vi "4 probe data v1.3.vi"() -> ()   [LabVIEW 2014]
uses:
  <vilib>/Analysis/baseanly.llb/Mean (DBL).vi
  <instrlib>/Keithley 24XX/Public/Data/Read (Single Point).vi
  <vilib>/MakerHub/LINX/Public/Peripherals/Analog/Analog Read 1 Chan.vi
  <instrlib>/Tektronix TDS 200 1000 2000 Series/Tektronix TDS 200 1000 2000 Series.lvlib
  <vilib>/MakerHub/LINX/LMH-LINX.lvlib
  <vilib>/Analysis/NI_AALBase.lvlib
  <instrlib>/Keithley 24XX/Keithley 24XX.lvlib
panel:
  out "Resistance-Time":sgl[](graph)
  out "Data IV Keithley":string
  in  "Data IV Keithley 2":path=path "c:/myfile.txt"
  out "IV Curve":cluster{sgl[], dbl[]}(graph)
  in  "Stop Voltage/Current":dbl=2.0
  in  "VISA resource name 2":refnum<visa-resource-name>="GPIB9::24::INSTR"
  in  "Serial Configuration 2":T1={"Baud Rate"=9600, "Parity"=0, "Data Bits"=8, "Stop Bits"=10, "Flow Control"=0} {"Flow Control" items=["None", "XON/XOFF", "RTS/CTS", "XON/XOFF & RTS/CTS", "DTR/DSR", "XON/XOFF & DTR/DSR"]; "Stop Bits" items=["1.0"=10, "1.5"=15, "2.0"=20]; "Data Bits" items=["7"=7, "8"=8]; "Parity" items=["None", "Odd", "Even", "Mark", "Space"]; "Baud Rate" items=["300"=300, "600"=600, "1200"=1200, "2400"=2400, "4800"=4800, "9600"=9600, "19200"=19200]}
  out "Voltage":sgl
  out "Current":sgl
  out "Resistance":sgl
  in  "Voltage Manual Range (1.0)":dbl=1.0
  in  "Current Manual Range (1.0)":dbl=1.0
  in  "Resistance Manual Range (1.0)":dbl=1.0
  in  "Enable Voltage Auto Range (T:Enable)":bool
  in  "Enable Current Auto Range (T:Enable)":bool=TRUE
  in  "Enable Resistance Auto Range (T:Enable)":bool
  in  "Compliance  Level (0.1)":dbl=1.0
  in  "Source Mode  (0: Voltage)":u16(ring) items=["Voltage", "Current"]
  in  "Step":dbl=1.0
  in  "current multiplier":dbl=1.0
  in  "Start Voltage/Current":dbl
  in  "Stop Button":bool
  out "Ard 4":dbl
  out "Ard 3":dbl
  out "Ard 2":dbl
  out "Ard 1":dbl
  out "Ard 0":dbl
  out "Data Ch4":string
  in  "Data Ch4":path=path "c:/myfile4.txt"
  out "Ard3-Osc4":cluster{"Y":dbl[], "Y":dbl[]}[](graph)
  out "Data Ch3":string
  in  "Data Ch3":path=path "c:/myfile3.txt"
  out "Ard2-Osc 3":cluster{"Y":dbl[], "Y":dbl[]}[](graph)
  out "Data Ch2":string
  in  "Data Ch2":path=path "c:/myfile2.txt"
  out "Ard1-Osc 2":cluster{"Y":dbl[], "Y":dbl[]}[](graph)
  out "Data Ch1":string
  in  "Data Ch1":path=path "c:/myfile1.txt"
  out "Ard0-Osc 1":cluster{"Y":dbl[], "Y":dbl[]}[](graph)
  out "Ch1":dbl
  out "Ch2":dbl
  out "Ch3":dbl
  out "Ch4":dbl
  out "Loop Rate (Hz)":u32
  out "Analog Data 4":dbl(graph)
  in  "AI Channel 4":u8=4
  in  "AI Channel 3":u8=3
  in  "AI Channel 2":u8=2
  in  "AI Channel 1":u8=1
  in  "AI Channel 0":u8
  in  "Serial Port":refnum<visa-resource-name>="COM6"
  in  "Channel 4 (3: Channel 4)":u16(ring)=3 items=["Channel 1", "Channel 2", "Channel 3", "Channel 4", "Math", "Reference A", "Reference B", "Reference C", "Reference D"]
  in  "Probe Attenuation 4 (0.1)":dbl=0.1
  in  "Vertical Coupling 4 (1: DC)":u16(ring)=1 items=["AC", "DC", "Ground"]
  in  "Channel 3 (2: Channel 3)":u16(ring)=2 items=["Channel 1", "Channel 2", "Channel 3", "Channel 4", "Math", "Reference A", "Reference B", "Reference C", "Reference D"]
  in  "Probe Attenuation 3 (0.1)":dbl=0.1
  in  "Vertical Coupling 3 (1: DC)":u16(ring)=1 items=["AC", "DC", "Ground"]
  in  "Channel 2 (1: Channel 2)":u16(ring)=1 items=["Channel 1", "Channel 2", "Channel 3", "Channel 4", "Math", "Reference A", "Reference B", "Reference C", "Reference D"]
  in  "Channel 1 (0: Channel 1)":u16(ring) items=["Channel 1", "Channel 2", "Channel 3", "Channel 4", "Math", "Reference A", "Reference B", "Reference C", "Reference D"]
  in  "Serial Configuration":T2={"Baud Rate"=9600, "Parity"=0, "Stop Bits"=10, "Flow Control"=2} {"Flow Control" items=["None", "XON/XOFF", "RTS/CTS", "XON/XOFF & RTS/CTS", "DTR/DSR", "XON/XOFF & DTR/DSR"]; "Stop Bits" items=["1.0"=10, "1.5"=15, "2.0"=20]; "Parity" items=["None", "Odd", "Even", "Mark", "Space"]; "Baud Rate" items=["300"=300, "600"=600, "1200"=1200, "2400"=2400, "4800"=4800, "9600"=9600, "19200"=19200]}
  in  "Probe Attenuation 2 (0.1)":dbl=0.1
  in  "Vertical Coupling 2 (1: DC)":u16(ring)=1 items=["AC", "DC", "Ground"]
  in  "Probe Attenuation 1 (0.1)":dbl=0.1
  in  "Vertical Coupling 1 (1: DC)":u16(ring)=1 items=["AC", "DC", "Ground"]
  in  "Timeout (10000 ms)":u32=500
  in  "VISA resource name":refnum<visa-resource-name>="USB0::0x0699::0x03A6::C044157::INSTR"
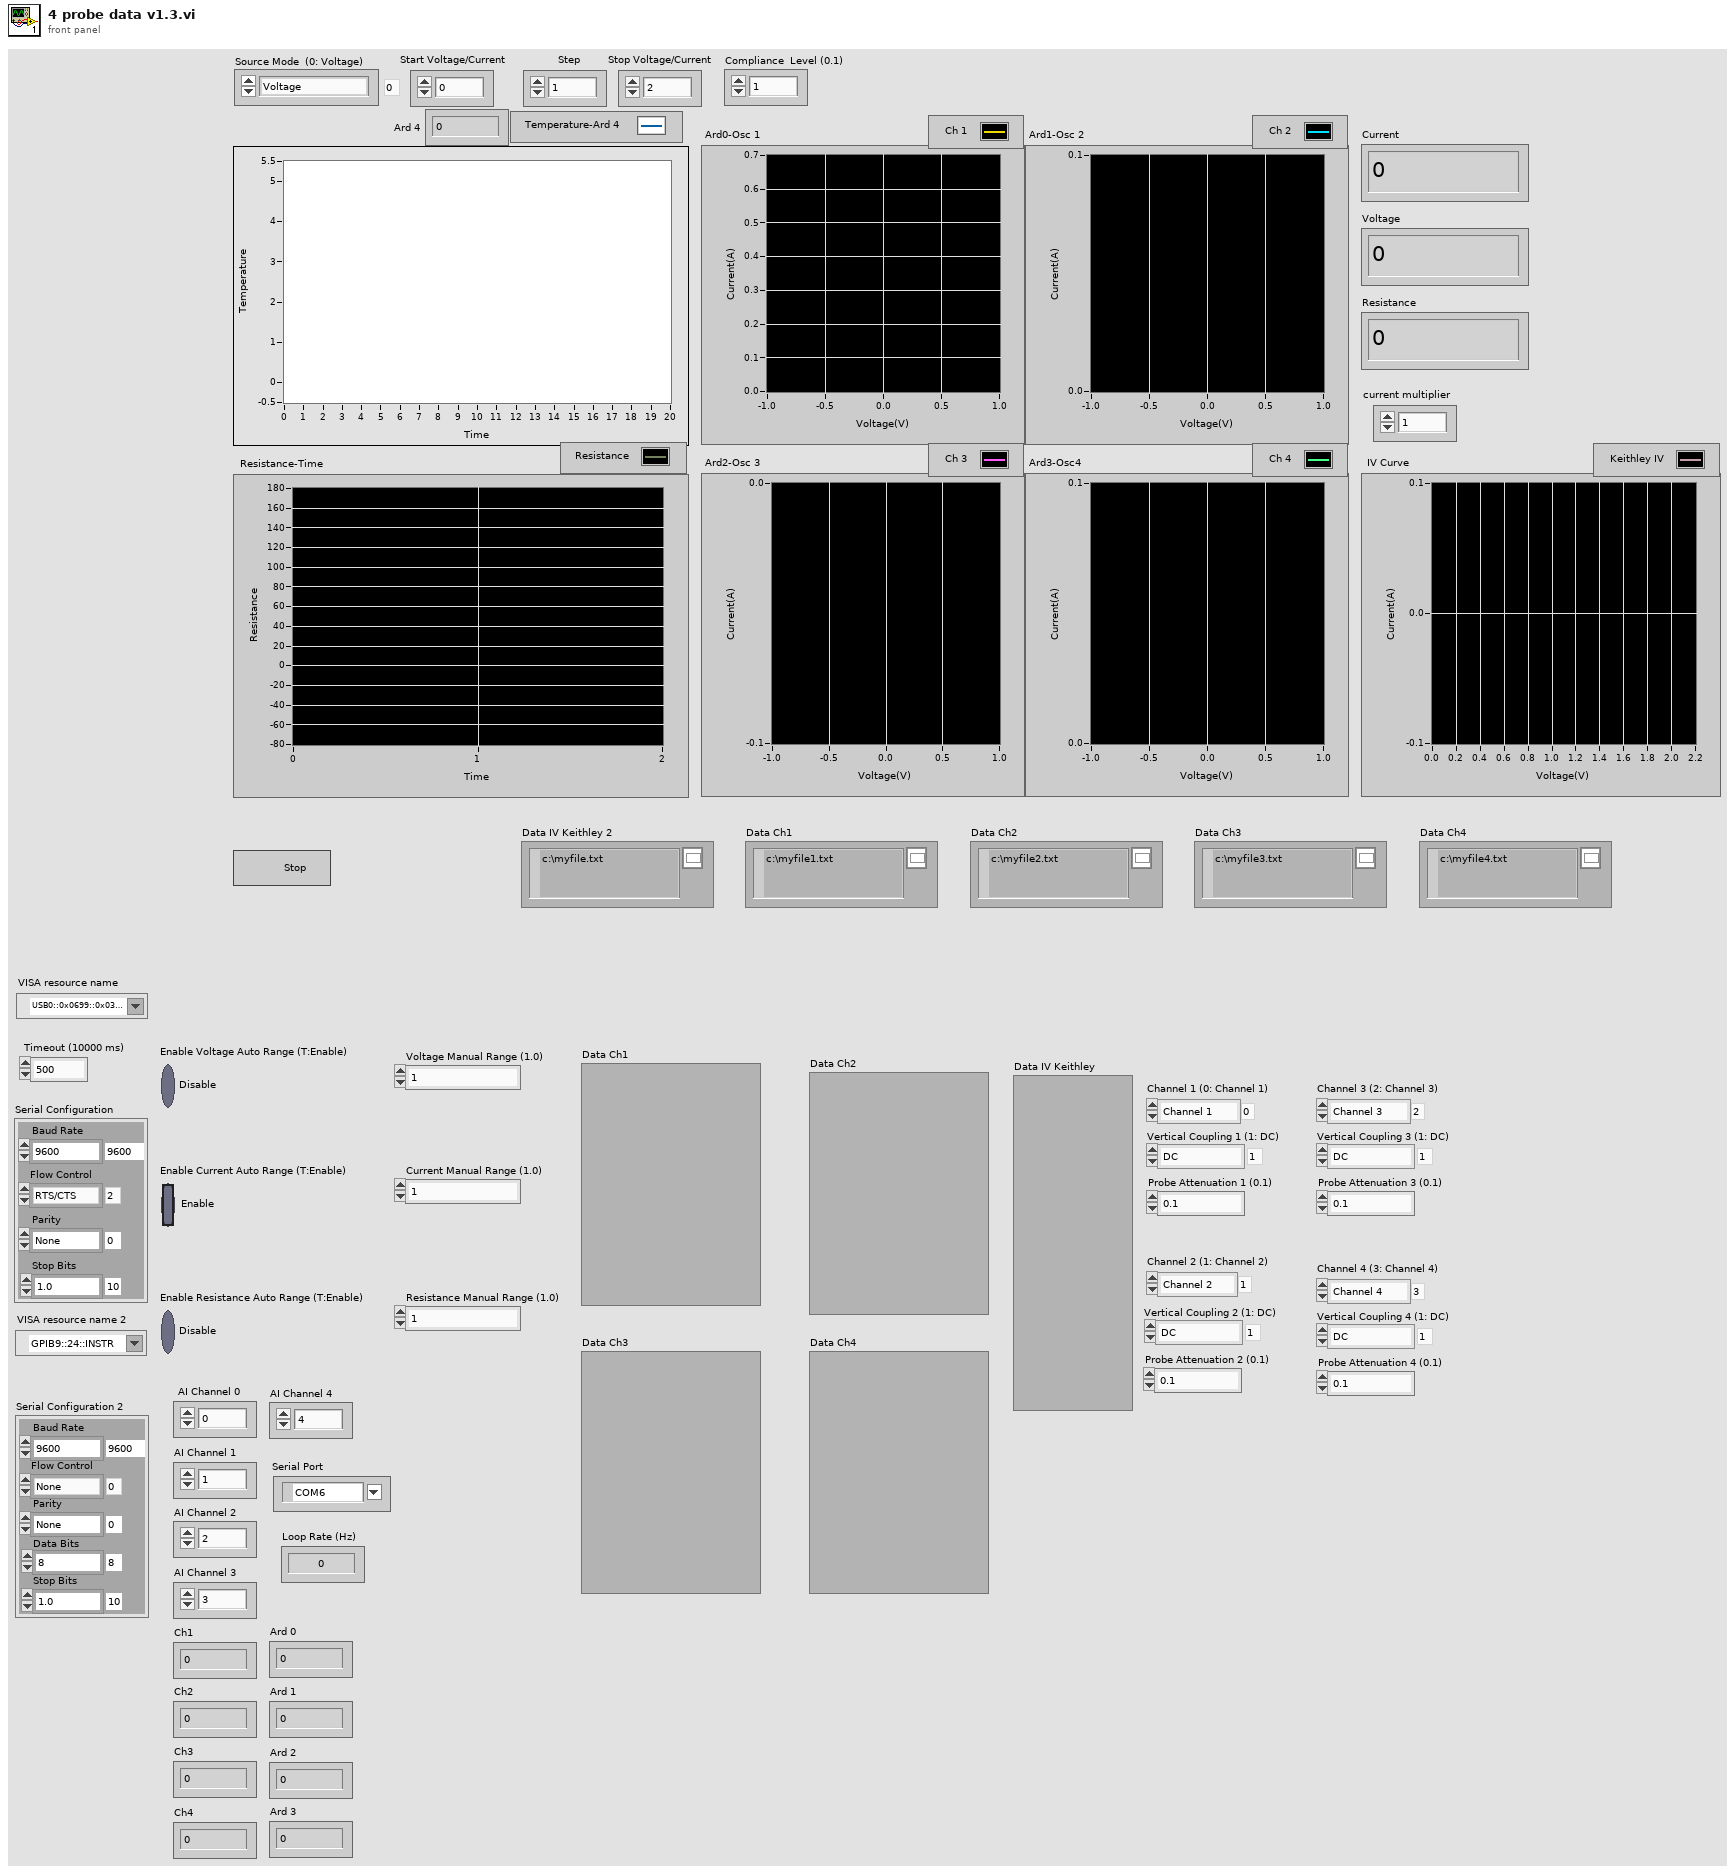
[diagram p1: front panel]
types:
  T1 = cluster{"Baud Rate":u32, "Parity":u16, "Data Bits":u16, "Stop Bits":u16, "Flow Control":u16}
  T2 = cluster{"Baud Rate":u32, "Parity":u16, "Stop Bits":u16, "Flow Control":u16}
  T3 = enum16{"open", "replace", "create", "open or create", "replace or create", "replace or create with confirmation"}
  T4 = typedef "LMH-LINX.lvlib/LINX Ref.ctl" = cluster{"Platform":T5, "Interface":T6, "LINX Device Config":T7}
  T5 = typedef "LMH-LINX.lvlib/Platform.ctl" = enum16{"LINX", "myRIO"}
  T6 = typedef "LMH-LINX.lvlib/Interface.ctl" = enum16{"Serial", "TCP"}
  T7 = typedef "LMH-LINX.lvlib/Device.lvlib/LINX Device Config.ctl" = cluster{"Interface":T6, "COM Port":refnum<visa-resource-name>, "TCP Configuration":T8, "Device Family":u8, "Device ID":u8, "Device Name":string, "TCP Ref":refnum<k5>, "Channels":T9}
  T8 = typedef "LMH-LINX.lvlib/Device.lvlib/TCP Config.ctl" = cluster{"IP Address":string, "Port":u16}
  T9 = typedef "LMH-LINX.lvlib/Channels.ctl" = cluster{"DI":u8[], "DO":u8[], "AI":u8[], "AO":u8[], "PWM":u8[], "QE":u8[], "UART":u8[], "I2C 2":u8[], "SPI":u8[], "CAN":u8[], "Servo":u8[], "AI Ref (V)":dbl, "AO Ref (V)":dbl, "AO Resolution (Bits)":u8}
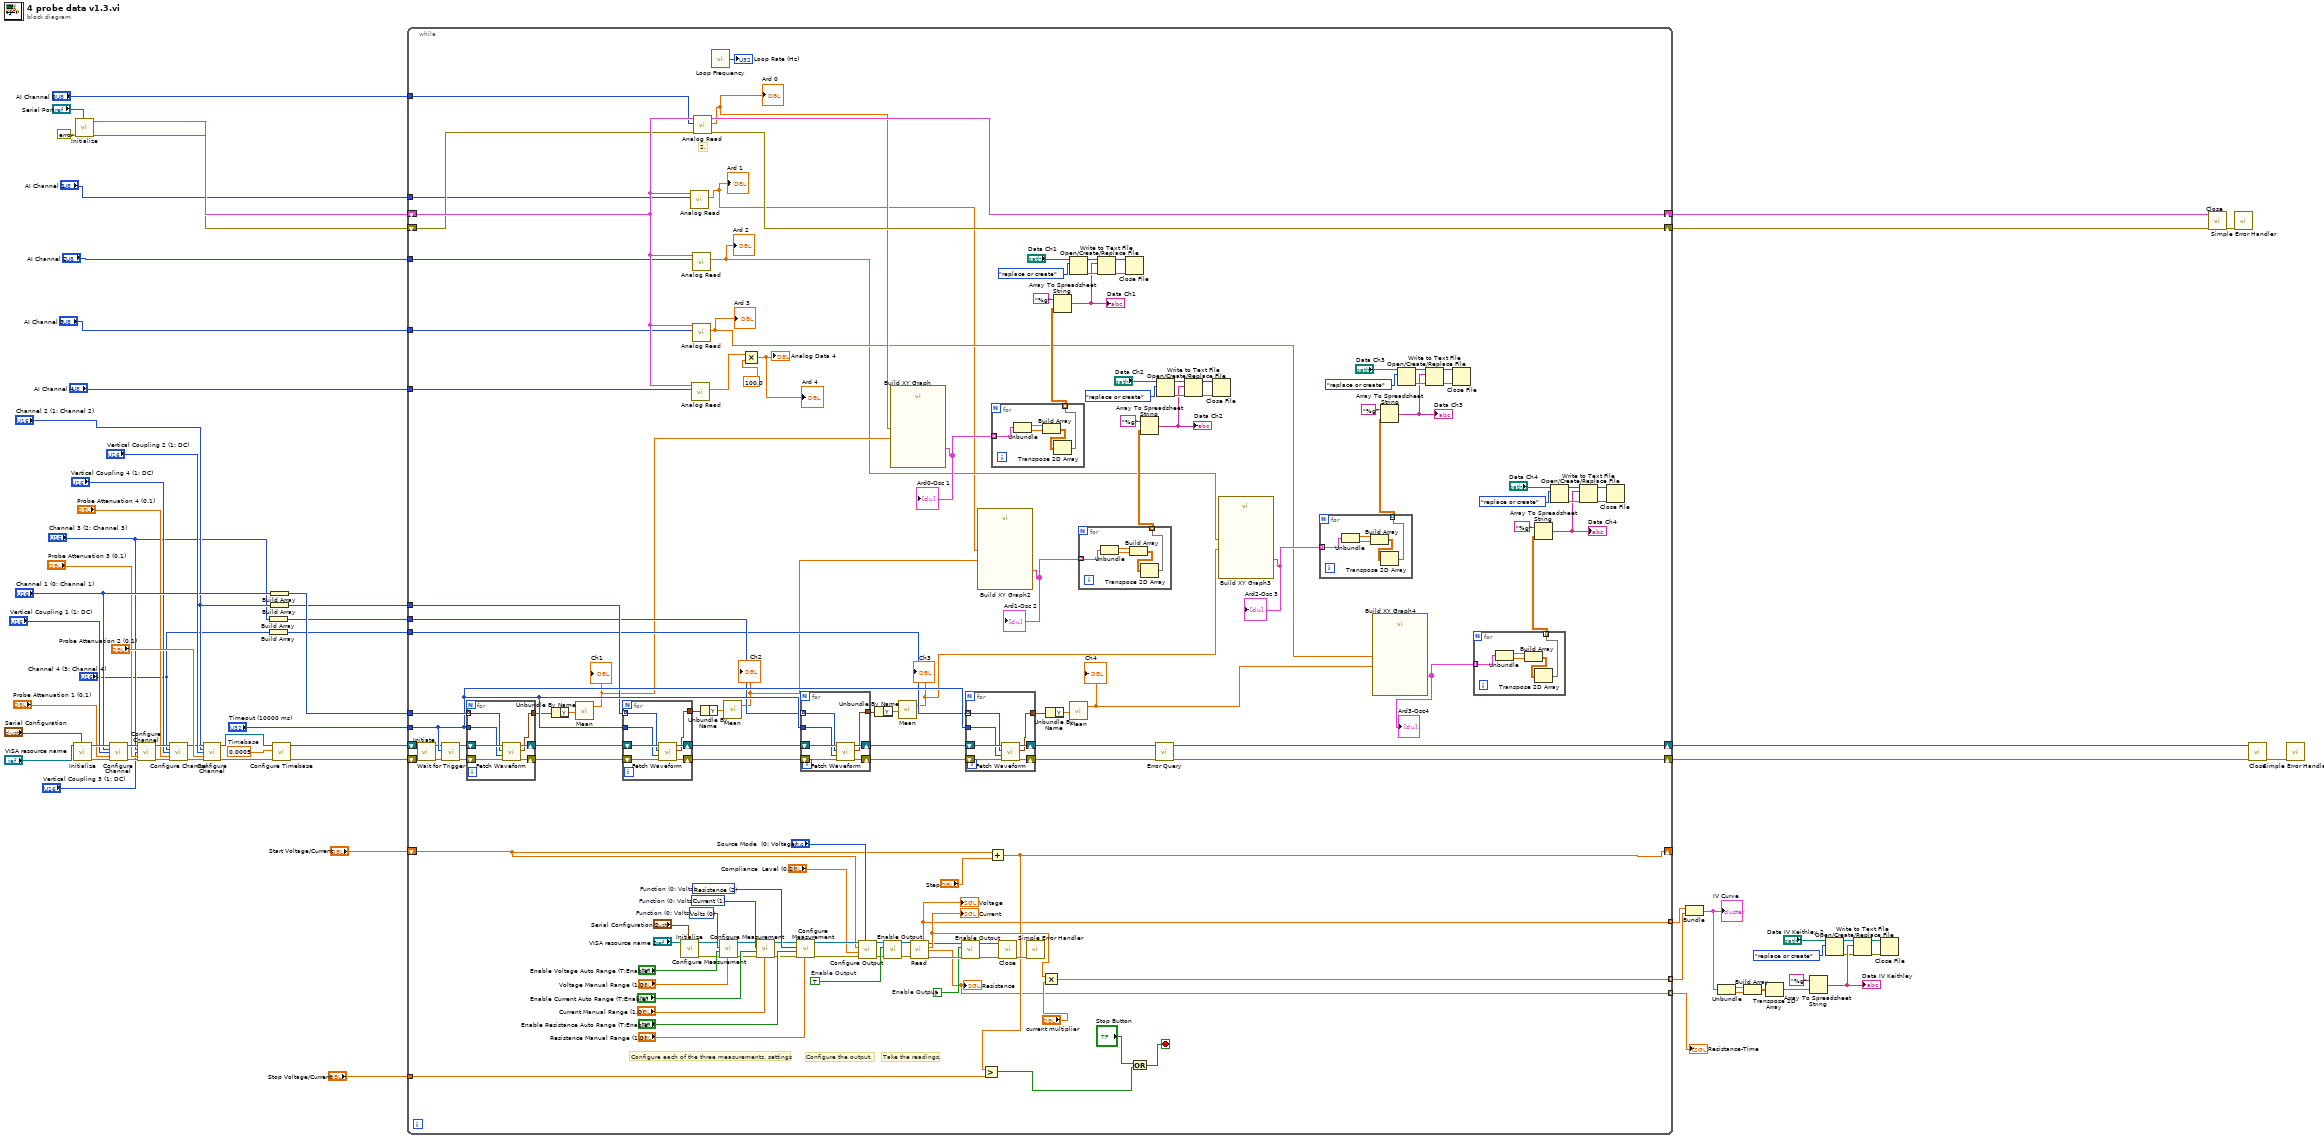
[diagram p0: block diagram]
diagram:
  w51 = 0.0005  # Timebase
  n1 = call <instrlib>:"Initialize.vi"("Serial Configuration"="Serial Configuration", "VISA resource name"="VISA resource name") -> ("error out"=w60:errorcluster, "VISA resource name out"=w61:refnum<visa-resource-name>)  [unwired: 3 in, 5 out]
  n2 = call <instrlib>:"Initialize.vi"("Serial Port"="Serial Port", "Error In"=errorcluster {"status"=FALSE, "code"=0, "source"=""}) -> ("Error Out"=w29:errorcluster, "LINX Ref"=w30:T4)  [unwired: 7 in, 1 out]
  n3 = call <instrlib>:"Configure Channel.vi"("VISA resource name"=w61, "Channel (0: Channel 1)"="Channel 1 (0: Channel 1)", "Vertical Coupling (1: DC)"="Vertical Coupling 1 (1: DC)", "Probe Attenuation (10: 10X)"="Probe Attenuation 1 (0.1)", "error in (no error)"=w60) -> ("VISA resource name out"=w46:refnum<visa-resource-name>, "error out"=w43:errorcluster)  [unwired: 4 in, 5 out]
  n4 = call <instrlib>:"Configure Channel.vi"("VISA resource name"=w46, "Channel (0: Channel 1)"="Channel 3 (2: Channel 3)", "Vertical Coupling (1: DC)"="Vertical Coupling 3 (1: DC)", "Probe Attenuation (10: 10X)"="Probe Attenuation 3 (0.1)", "error in (no error)"=w43) -> ("VISA resource name out"=w45:refnum<visa-resource-name>, "error out"=w42:errorcluster)  [unwired: 4 in, 5 out]
  n5 = call <instrlib>:"Configure Channel.vi"("VISA resource name"=w45, "Channel (0: Channel 1)"="Channel 4 (3: Channel 4)", "Vertical Coupling (1: DC)"="Vertical Coupling 4 (1: DC)", "Probe Attenuation (10: 10X)"="Probe Attenuation 4 (0.1)", "error in (no error)"=w42) -> ("VISA resource name out"=w44:refnum<visa-resource-name>, "error out"=w41:errorcluster)  [unwired: 4 in, 5 out]
  n6 = call <instrlib>:"Configure Channel.vi"("VISA resource name"=w44, "Channel (0: Channel 1)"="Channel 2 (1: Channel 2)", "Vertical Coupling (1: DC)"="Vertical Coupling 2 (1: DC)", "Probe Attenuation (10: 10X)"="Probe Attenuation 2 (0.1)", "error in (no error)"=w41) -> ("VISA resource name out"=w59:refnum<visa-resource-name>, "error out"=w58:errorcluster)  [unwired: 4 in, 5 out]
  n7 = Build Array("Channel 3 (2: Channel 3)") -> (w32:u16[])
  n8 = Build Array("Channel 4 (3: Channel 4)") -> (w31:u16[])
  n9 = Build Array("Channel 1 (0: Channel 1)") -> (w50:u16[])
  n10 = Build Array("Channel 2 (1: Channel 2)") -> (w35:u16[])
  n11 = call <instrlib>:"Configure Timebase.vi"("error in (no error)"=w58, "Timebase (0.0005 s)"=w51, "VISA resource name"=w59) -> ("error out"=w56:errorcluster, "VISA resource name out"=w57:refnum<visa-resource-name>)  [unwired: 1 in, 6 out]
  n12 = while {
    tunnel: w50 -> [w195]
    tunnel: "Timeout (10000 ms)" -> [w194]
    tunnel: w35 -> [w193]
    tunnel: w32 -> [w192]
    tunnel: w31 -> [w191]
    tunnel: "AI Channel 0" -> [w166]
    tunnel: "AI Channel 1" -> [w165]
    tunnel: "AI Channel 2" -> [w164]
    tunnel: "AI Channel 3" -> [w163]
    tunnel: "AI Channel 4" -> [w162]
    shift-right: [w199] -> w63
    shift-left: w57 -> [w197]
    shift-right: [w198] -> w62
    shift-left: w56 -> [w196]
    shift-right: [w168] -> w28
    shift-left: w30 -> [w170]
    shift-right: [w167] -> w27
    shift-left: w29 -> [w169]
    tunnel: "Stop Voltage/Current" -> [w74]
    shift-right: [w72] -> _
    shift-left: "Start Voltage/Current" -> [w73]
    tunnel: [w68] -> w3 mode=indexing
    tunnel: [w67] -> w2 mode=indexing
    tunnel: [w66] -> w1 mode=indexing
    stop <- w69 stop-if-true
    w103 = TRUE  # Enable Output
    w93 = FALSE  # Enable Output
    w86 = u16 2 items=["Volts", "Current", "Resistance"]  # Function (0: Volts)
    w85 = u16 1 items=["Volts", "Current", "Resistance"]  # Function (0: Volts)
    w84 = u16 0 items=["Volts", "Current", "Resistance"]  # Function (0: Volts)
    # "Take the readings."
    # "Configure the output."
    # "Configure each of the three measurements. settings"
    # "2."
    n13 = call <instrlib>:"Initiate.vi"("error in (no error)"=w196, "VISA resource name"=w197) -> ("error out"=w187:errorcluster, "VISA resource name out"=w190:refnum<visa-resource-name>)  [unwired: 8 out]
    n14 = call <instrlib>:"Wait for Trigger.vi"("error in (no error)"=w187, "Timeout (10000 ms)"=w194, "VISA resource name"=w190) -> ("error out"=w188:errorcluster, "VISA resource name out"=w189:refnum<visa-resource-name>)  [unwired: 7 out]
    n15 = for {
      shift-right: [w246] -> w185
      shift-left: w188 -> [w244]
      tunnel: w195 -> [w242] mode=indexing
      tunnel: w194 -> [w243]
      shift-right: [w247] -> w186
      shift-left: w189 -> [w245]
      tunnel: [w241] -> w178
      n16 = call <instrlib>:"Fetch Waveform.vi"("error in (no error)"=w244, "Timeout (10000 ms)"=w243, "Source (0: Channel 1)"=w242, "VISA resource name"=w245) -> ("error out"=w246:errorcluster, "Waveform Data"=w241:waveform(dbl), "VISA resource name out"=w247:refnum<visa-resource-name>)  [unwired: 2 in, 3 out]
    }
    n17 = Unbundle By Name(w178) -> ("Y"=w177:dbl[])
    n18 = call-poly <vilib>:"Mean.vi"("X"=w177) -> ("mean"=w148:dbl)  [unwired: 1 out]
    "Ch1" <- w148
    n19 = for {
      shift-right: [w239] -> w179
      shift-left: w185 -> [w237]
      tunnel: w193 -> [w235] mode=indexing
      tunnel: w194 -> [w236]
      shift-right: [w240] -> w180
      shift-left: w186 -> [w238]
      tunnel: [w234] -> w174
      n20 = call <instrlib>:"Fetch Waveform.vi"("error in (no error)"=w237, "Timeout (10000 ms)"=w236, "Source (0: Channel 1)"=w235, "VISA resource name"=w238) -> ("error out"=w239:errorcluster, "Waveform Data"=w234:waveform(dbl), "VISA resource name out"=w240:refnum<visa-resource-name>)  [unwired: 2 in, 3 out]
    }
    n21 = call <instrlib>:"Initialize.vi"("Serial Configuration"="Serial Configuration 2", "VISA resource name"="VISA resource name 2") -> ("error out"=w79:errorcluster, "VISA resource name out"=w78:refnum<visa-resource-name>)  [unwired: 8 in]
    n22 = call-poly <vilib>:"Analog Read.vi"("Analog Channel"=w165, "LINX Resource"=w170) -> ("AI Value"=w110:dbl)  [unwired: 6 in, 3 out]
    "Ard 1" <- w110
    n23 = call-poly <vilib>:"Analog Read.vi"("Analog Channel"=w162, "LINX Resource"=w170) -> ("AI Value"=w160:dbl)  [unwired: 6 in, 3 out]
    n24 = call-poly <vilib>:"Analog Read.vi"("Analog Channel"=w164, "LINX Resource"=w170) -> ("AI Value"=w111:dbl)  [unwired: 6 in, 3 out]
    "Ard 2" <- w111
    n25 = call-poly <vilib>:"Analog Read.vi"("Analog Channel"=w163, "LINX Resource"=w170) -> ("AI Value"=w112:dbl)  [unwired: 6 in, 3 out]
    "Ard 3" <- w112
    n26 = call-poly <vilib>:"Analog Read.vi"("Error In"=w169, "Analog Channel"=w166, "LINX Resource"=w170) -> ("Error Out"=w167:errorcluster, "AI Value"=w114:dbl, "LINX Resource"=w168:T4)  [unwired: 5 in, 1 out]
    "Ard 0" <- w114
    n27 = Unbundle By Name(w174) -> ("Y"=w173:dbl[])
    n28 = call <vilib>:"Loop Frequency.vi"() -> ("Loop Rate (Hz)"=→"Loop Rate (Hz)":u32)
    n29 = call <instrlib>:"Configure Measurement.vi"("Manual Range (1.0)"="Voltage Manual Range (1.0)", "error in (no error)"=w79, "Enable Auto Range (T:Enable)"="Enable Voltage Auto Range (T:Enable)", "Function (0: Volts)"=w84, "VISA resource name"=w78) -> ("error out"=w81:errorcluster, "VISA resource name out"=w80:refnum<visa-resource-name>)  [unwired: 5 in]
    n30 = call-poly <vilib>:"Mean.vi"("X"=w173) -> ("mean"=w137:dbl)  [unwired: 1 out]
    "Ch2" <- w137
    n31 = Multiply(x=w160, y=100.0) -> (x*y=→"Analog Data 4" →"Ard 4":dbl)
    n32 = call <instrlib>:"Configure Measurement.vi"("Manual Range (1.0)"="Current Manual Range (1.0)", "error in (no error)"=w81, "Enable Auto Range (T:Enable)"="Enable Current Auto Range (T:Enable)", "Function (0: Volts)"=w85, "VISA resource name"=w80) -> ("error out"=w82:errorcluster, "VISA resource name out"=w83:refnum<visa-resource-name>)  [unwired: 5 in]
    n33 = call <instrlib>:"Configure Measurement.vi"("Manual Range (1.0)"="Resistance Manual Range (1.0)", "error in (no error)"=w82, "Enable Auto Range (T:Enable)"="Enable Resistance Auto Range (T:Enable)", "Function (0: Volts)"=w86, "VISA resource name"=w83) -> ("error out"=w104:errorcluster, "VISA resource name out"=w105:refnum<visa-resource-name>)  [unwired: 5 in]
    n34 = for {
      shift-right: [w232] -> w183
      shift-left: w179 -> [w230]
      tunnel: w192 -> [w228] mode=indexing
      tunnel: w194 -> [w229]
      shift-right: [w233] -> w184
      shift-left: w180 -> [w231]
      tunnel: [w227] -> w175
      n35 = call <instrlib>:"Fetch Waveform.vi"("error in (no error)"=w230, "Timeout (10000 ms)"=w229, "Source (0: Channel 1)"=w228, "VISA resource name"=w231) -> ("error out"=w232:errorcluster, "Waveform Data"=w227:waveform(dbl), "VISA resource name out"=w233:refnum<visa-resource-name>)  [unwired: 2 in, 3 out]
    }
    n36 = call <instrlib>:"Configure Output.vi"("Source Mode  (0: Voltage)"="Source Mode  (0: Voltage)", "error in (no error)"=w104, "Compliance  Level (0.1)"="Compliance  Level (0.1)", "Output Level (0)"=w73, "VISA resource name"=w105) -> ("error out"=w102:errorcluster, "VISA resource name out"=w101:refnum<visa-resource-name>)  [unwired: 5 in]
    n37 = Unbundle By Name(w175) -> ("Y"=w172:dbl[])
    n38 = call <instrlib>:"Enable Output.vi"("error in (no error)"=w102, "Enable Output (T: Enable)"=w103, "VISA resource name"=w101) -> ("error out"=w99:errorcluster, "VISA resource name out"=w100:refnum<visa-resource-name>)  [unwired: 7 in]
    n39 = call "Build XY Graph"("Y Input"=w148, "X Input"=w114) -> ("XY Graph"=w149:cluster{"Y":dbl[], "Y":dbl[]}[])  [unwired: 8 in, 1 out]
    "Ard0-Osc 1" <- w149
    n40 = call-poly <vilib>:"Mean.vi"("X"=w172) -> ("mean"=w126:dbl)  [unwired: 1 out]
    "Ch3" <- w126
    n41 = call-poly <instrlib>:"Read.vi"("VISA resource name"=w100, "error in (no error)"=w99) -> ("Voltage"=w67:sgl, "VISA resource name out"=w98:refnum<visa-resource-name>, "Current"=w108:sgl, "Resistance"=w66:sgl, "error out"=w97:errorcluster)  [unwired: 7 in, 2 out]
    "Voltage" <- w67
    "Current" <- w108
    "Resistance" <- w66
    n42 = call <instrlib>:"Enable Output.vi"("error in (no error)"=w97, "Enable Output (T: Enable)"=w93, "VISA resource name"=w98) -> ("error out"=w96:errorcluster, "VISA resource name out"=w95:refnum<visa-resource-name>)  [unwired: 7 in]
    n43 = for {
      shift-right: [w225] -> w181
      shift-left: w183 -> [w223]
      tunnel: w191 -> [w221] mode=indexing
      tunnel: w194 -> [w222]
      shift-right: [w226] -> w182
      shift-left: w184 -> [w224]
      tunnel: [w220] -> w176
      n44 = call <instrlib>:"Fetch Waveform.vi"("error in (no error)"=w223, "Timeout (10000 ms)"=w222, "Source (0: Channel 1)"=w221, "VISA resource name"=w224) -> ("error out"=w225:errorcluster, "Waveform Data"=w220:waveform(dbl), "VISA resource name out"=w226:refnum<visa-resource-name>)  [unwired: 2 in, 3 out]
    }
    n45 = call "Build XY Graph2"("Y Input"=w137, "X Input"=w110) -> ("XY Graph"=w138:cluster{"Y":dbl[], "Y":dbl[]}[])  [unwired: 8 in, 1 out]
    "Ard1-Osc 2" <- w138
    n46 = Add(x=w73, y="Step") -> (x+y=w72:dbl)
    n47 = Greater?(x=w72, y=w74) -> (0:w71:bool)
    n48 = for {
      tunnel: w149 -> [w219] mode=indexing
      tunnel: [w215] -> w150 mode=indexing
      n49 = Unbundle(w219) -> ("Y"=w218:dbl[], "Y"=w217:dbl[])
      n50 = Build Array(w218, w217) -> (w216:dbl[][])
      n51 = Transpose 2D Array(2D array=w216) -> (transposed array=w215:dbl[][])
    }
    n52 = call <instrlib>:"Close.vi"("error in (no error)"=w96, "VISA resource name"=w95) -> ("error out"=w75:errorcluster)  [unwired: 9 in]
    n53 = call <vilib>:"Simple Error Handler.vi"("error in (no error)"=w75) -> ()  [unwired: 4 in, 5 out]
    n54 = Multiply(x=w108, y="current multiplier") -> (x*y=w68:dbl)
    n55 = Unbundle By Name(w176) -> ("Y"=w171:dbl[])
    n56 = Array To Spreadsheet String(array=w150, 3:"%g" ("format string")) -> (spreadsheet string=w151:string)  [unwired: 1 in]
    "Data Ch1" <- w151
    n57 = Open/Create/Replace File(file path (use dialog)="Data Ch1", operation (0:open)=T3."replace or create") -> (refnum out=w153:refnum<file>, error out=w158:errorcluster)  [unwired: 4 in, 1 out]
    n58 = call-poly <vilib>:"Mean.vi"("X"=w171) -> ("mean"=w115:dbl)  [unwired: 1 out]
    "Ch4" <- w115
    n59 = for {
      tunnel: w138 -> [w214] mode=indexing
      tunnel: [w210] -> w139 mode=indexing
      n60 = Unbundle(w214) -> ("Y"=w213:dbl[], "Y"=w212:dbl[])
      n61 = Build Array(w213, w212) -> (w211:dbl[][])
      n62 = Transpose 2D Array(2D array=w211) -> (transposed array=w210:dbl[][])
    }
    n63 = Write to Text File(file (use dialog)=w153, text=w151, error in=w158) -> (refnum out=w156:refnum<file>, error out=w157:errorcluster)  [unwired: 2 out]
    n64 = Close File(refnum=w156, error in=w157) -> ()  [unwired: 2 out]
    n65 = Or(x="Stop Button", y=w71) -> (x .or. y?=w69:bool)
    n66 = Array To Spreadsheet String(array=w139, 3:"%g" ("format string")) -> (spreadsheet string=w140:string)  [unwired: 1 in]
    "Data Ch2" <- w140
    n67 = call <instrlib>:"Error Query.vi"("error in (no error)"=w181, "VISA resource name"=w182) -> ("error out"=w198:errorcluster, "VISA resource name out"=w199:refnum<visa-resource-name>)  [unwired: 8 out]
    n68 = Open/Create/Replace File(file path (use dialog)="Data Ch2", operation (0:open)=T3."replace or create") -> (refnum out=w142:refnum<file>, error out=w147:errorcluster)  [unwired: 4 in, 1 out]
    n69 = Write to Text File(file (use dialog)=w142, text=w140, error in=w147) -> (refnum out=w145:refnum<file>, error out=w146:errorcluster)  [unwired: 2 out]
    n70 = Close File(refnum=w145, error in=w146) -> ()  [unwired: 2 out]
    n71 = call "Build XY Graph3"("Y Input"=w126, "X Input"=w111) -> ("XY Graph"=w127:cluster{"Y":dbl[], "Y":dbl[]}[])  [unwired: 8 in, 1 out]
    "Ard2-Osc 3" <- w127
    n72 = for {
      tunnel: w127 -> [w209] mode=indexing
      tunnel: [w205] -> w128 mode=indexing
      n73 = Unbundle(w209) -> ("Y"=w208:dbl[], "Y"=w207:dbl[])
      n74 = Build Array(w208, w207) -> (w206:dbl[][])
      n75 = Transpose 2D Array(2D array=w206) -> (transposed array=w205:dbl[][])
    }
    n76 = call "Build XY Graph4"("Y Input"=w115, "X Input"=w112) -> ("XY Graph"=w116:cluster{"Y":dbl[], "Y":dbl[]}[])  [unwired: 8 in, 1 out]
    "Ard3-Osc4" <- w116
    n77 = Array To Spreadsheet String(array=w128, 3:"%g" ("format string")) -> (spreadsheet string=w129:string)  [unwired: 1 in]
    "Data Ch3" <- w129
    n78 = Open/Create/Replace File(file path (use dialog)="Data Ch3", operation (0:open)=T3."replace or create") -> (refnum out=w131:refnum<file>, error out=w136:errorcluster)  [unwired: 4 in, 1 out]
    n79 = Write to Text File(file (use dialog)=w131, text=w129, error in=w136) -> (refnum out=w134:refnum<file>, error out=w135:errorcluster)  [unwired: 2 out]
    n80 = Close File(refnum=w134, error in=w135) -> ()  [unwired: 2 out]
    n81 = for {
      tunnel: w116 -> [w204] mode=indexing
      tunnel: [w200] -> w117 mode=indexing
      n82 = Unbundle(w204) -> ("Y"=w203:dbl[], "Y"=w202:dbl[])
      n83 = Build Array(w203, w202) -> (w201:dbl[][])
      n84 = Transpose 2D Array(2D array=w201) -> (transposed array=w200:dbl[][])
    }
    n85 = Array To Spreadsheet String(array=w117, 3:"%g" ("format string")) -> (spreadsheet string=w118:string)  [unwired: 1 in]
    "Data Ch4" <- w118
    n86 = Open/Create/Replace File(file path (use dialog)="Data Ch4", operation (0:open)=T3."replace or create") -> (refnum out=w120:refnum<file>, error out=w125:errorcluster)  [unwired: 4 in, 1 out]
    n87 = Write to Text File(file (use dialog)=w120, text=w118, error in=w125) -> (refnum out=w123:refnum<file>, error out=w124:errorcluster)  [unwired: 2 out]
    n88 = Close File(refnum=w123, error in=w124) -> ()  [unwired: 2 out]
  }
  "Resistance-Time" <- w1
  n89 = Bundle(w2, w3) -> (w12:cluster{sgl[], dbl[]})  [unwired: 1 out]
  "IV Curve" <- w12
  n90 = Unbundle(w12) -> (w13:sgl[], w14:dbl[])
  n91 = Build Array(w13, w14) -> (w15:dbl[][])
  n92 = Transpose 2D Array(2D array=w15) -> (transposed array=w17:dbl[][])
  n93 = Array To Spreadsheet String(array=w17, 3:"%g" ("format string")) -> (spreadsheet string=w18:string)  [unwired: 1 in]
  "Data IV Keithley" <- w18
  n94 = Open/Create/Replace File(file path (use dialog)="Data IV Keithley 2", operation (0:open)=T3."replace or create") -> (refnum out=w11:refnum<file>, error out=w6:errorcluster)  [unwired: 4 in, 1 out]
  n95 = Write to Text File(file (use dialog)=w11, text=w18, error in=w6) -> (refnum out=w8:refnum<file>, error out=w7:errorcluster)  [unwired: 2 out]
  n96 = Close File(refnum=w8, error in=w7) -> ()  [unwired: 2 out]
  n97 = call <instrlib>:"Close.vi"("Error In"=w27, "LINX Resource"=w28) -> ("Error Out"=w25:errorcluster)  [unwired: 8 in, 1 out]
  n98 = call <vilib>:"Simple Error Handler.vi"("error in (no error)"=w25) -> ()  [unwired: 4 in, 5 out]
  n99 = call <instrlib>:"Close.vi"("error in (no error)"=w62, "VISA resource name"=w63) -> ("error out"=w64:errorcluster)  [unwired: 9 out]
  n100 = call <vilib>:"Simple Error Handler.vi"("error in (no error)"=w64) -> ()  [unwired: 1 in, 8 out]
